vi "DMAWrites.vi"(10 "EncoderTimers":T1[](array[typedef])=[{"Period"=0.0, "Count"=0, "Stopped"=FALSE}, {"Period"=0.0, "Count"=0, "Stopped"=FALSE}, {"Period"=0.0, "Count"=0, "Stopped"=FALSE}, {"Period"=0.0, "Count"=0, "Stopped"=FALSE}, {"Period"=0.0, "Count"=0, "Stopped"=FALSE}, {"Period"=0.0, "Count"=0, "Stopped"=FALSE}, {"Period"=0.0, "Count"=0, "Stopped"=FALSE}, {"Period"=0.0, "Count"=0, "Stopped"=FALSE}], 11 "Encoders":T2[](array[typedef])=[{"Direction"=FALSE, "Value"=0.0}, {"Direction"=FALSE, "Value"=0.0}, {"Direction"=FALSE, "Value"=0.0}, {"Direction"=FALSE, "Value"=0.0}, {"Direction"=FALSE, "Value"=0.0}, {"Direction"=FALSE, "Value"=0.0}, {"Direction"=FALSE, "Value"=0.0}]) -> ()   [LabVIEW 2019]
uses:
  Helpers/CountingOutput.ctl
  Helpers/TimerOutput.ctl
panel:
  in  "CounterTimers":T1[](array[typedef])=[{"Period"=0.0, "Count"=0, "Stopped"=FALSE}, {"Period"=0.0, "Count"=0, "Stopped"=FALSE}, {"Period"=0.0, "Count"=0, "Stopped"=FALSE}, {"Period"=0.0, "Count"=0, "Stopped"=FALSE}, {"Period"=0.0, "Count"=0, "Stopped"=FALSE}, {"Period"=0.0, "Count"=0, "Stopped"=FALSE}, {"Period"=0.0, "Count"=0, "Stopped"=FALSE}, {"Period"=0.0, "Count"=0, "Stopped"=FALSE}]
  in  "Counters":T2[](array[typedef])=[{"Direction"=FALSE, "Value"=0.0}, {"Direction"=FALSE, "Value"=0.0}, {"Direction"=FALSE, "Value"=0.0}, {"Direction"=FALSE, "Value"=0.0}, {"Direction"=FALSE, "Value"=0.0}, {"Direction"=FALSE, "Value"=0.0}, {"Direction"=FALSE, "Value"=0.0}, {"Direction"=FALSE, "Value"=0.0}]
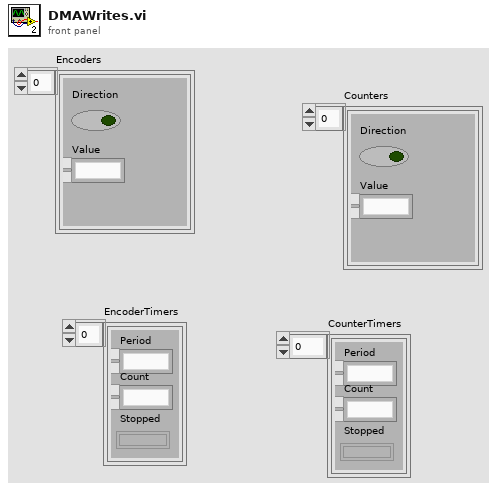
[diagram p1: front panel]
types:
  T1 = typedef "TimerOutput.ctl" = cluster{"Period":fxp<+,24,25>, "Count":i16, "Stopped":bool}
  T2 = typedef "CountingOutput.ctl" = cluster{"Direction":bool, "Value":fxp<+/-,31,31>}
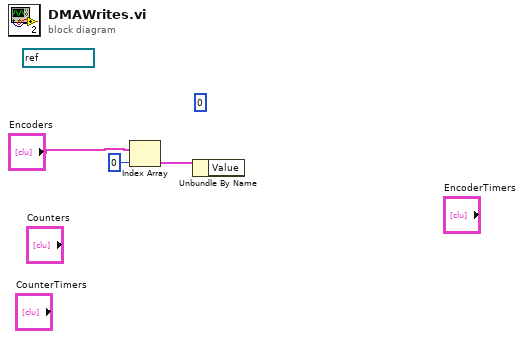
[diagram p0: block diagram]
diagram:
  (unwired) 0 ("Timeout")
  (unwired) refnum<k21> "RioDMA" ("FIFO In")
  n1 = Index Array(array="Encoders", index=0) -> (element=w1:T2)
  n2 = Unbundle By Name(w1) -> ()  [unwired: 1 out]
